vi "Friendly Name.vi"(8 "error in (no error)":errorcluster, 11 "DeployTCPResource in":refnum<class "TCPResource.lvclass">) -> (0 "error out":errorcluster, 2 "Friendly Name":string, 3 "DeployTCPResource out":refnum<class "TCPResource.lvclass">)   [LabVIEW 2020, in "PicoG-Core.lvlib" / "TCPResource.lvclass"]
uses:
  TCPResource.lvclass
  TCPResource.lvclass/TCPResource.ctl
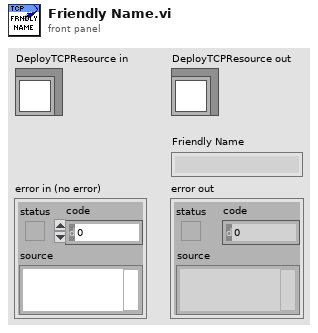
[diagram p1: front panel]
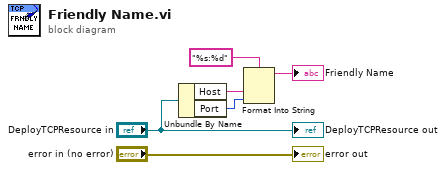
[diagram p0: block diagram]
diagram:
  n1 = Unbundle By Name("DeployTCPResource in") -> ("Host"=w4:string, "Port"=w3:u16)
  n2 = Format Into String(format string="%s:%d", w4, w3) -> (resulting string=→"Friendly Name":string)  [unwired: 2 in, 1 out]
  "error out" <- "error in (no error)"
  "DeployTCPResource out" <- "DeployTCPResource in"
